vi "题目5.vi"() -> ()   [LabVIEW 2017]
panel:
  in  "分数":i32
  out "警告":bool
  out "通过":bool
  out "恭喜":bool
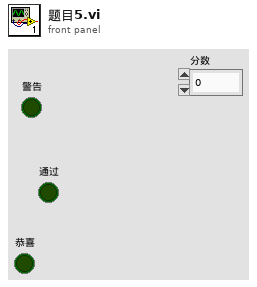
[diagram p1: front panel]
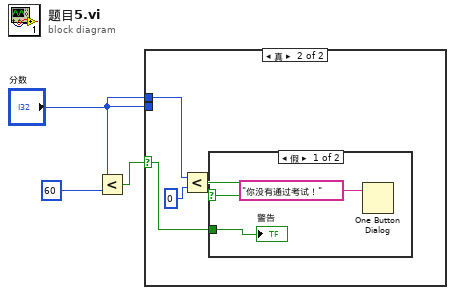
[diagram p0: block diagram]
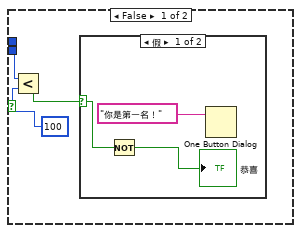
[diagram p2: hidden frame]
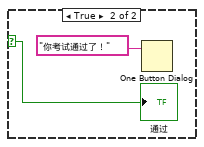
[diagram p3: hidden frame]
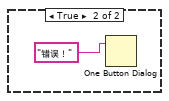
[diagram p4: hidden frame]
diagram:
  n1 = Less?(x="分数", y=60) -> (x < y?=w3:bool)
  n2 = case shown="真" w3 {
    selector: w3 -> [_ w12]
    tunnel: "分数" -> [w4 _]
    tunnel: "分数" -> [_ w14]
    frame False {
      n3 = Less?(x=w4, y=100) -> (x < y?=w6:bool)
      n4 = case shown="假" w6 {
        selector: w6 -> [w8 w10]
        frame False {
          n5 = Not(x=w8) -> (.not. x?=→"恭喜":bool)
          n6 = One Button Dialog(message="你是第一名！") -> ()  [unwired: 1 in, 1 out]
        }
        frame True {
          n7 = One Button Dialog(message="你考试通过了！") -> ()  [unwired: 1 in, 1 out]
          "通过" <- w10
        }
      }
    }
    frame True {
      n8 = Less?(x=w14, y=0) -> (x < y?=w15:bool)
      n9 = case shown="假" w15 {
        tunnel: w12 -> [w16 _]
        frame False {
          n10 = One Button Dialog(message="你没有通过考试！") -> ()  [unwired: 1 in, 1 out]
          "警告" <- w16
        }
        frame True {
          n11 = One Button Dialog(message="错误！") -> ()  [unwired: 1 in, 1 out]
        }
      }
    }
  }
